vi "Finish.vi"   [LabVIEW 2017]
doc: "This VI is called just before exiting. It is expected to close I/O refnum, save collected data, etc."
uses:
  <vilib>/Rock Robotics/WPI/Utilities/WPI_GetSetVariantRefNum.vi
types:
  T1 = typedef "WPI_MotorControlDeviceRef.ctl" = cluster{"DeviceStatus":errorcluster, "Type":T2, "PWM":cluster{"PWM Channel":T3, "DeadBand":T4}, "CAN":cluster{"Device Number":u8, "SetOutput VI Ref":variant, "GetOutput VI Ref":variant, "Enable VI Ref":variant, "Disable VI Ref":variant, "Data":variant}, "Invert":bool, "DIO PWM":cluster{"PWM \"Enable\" Channel":T3, "DIOChannel":T5, "PWM Rate":dbl}}
  T2 = typedef "WPI_MotorControlType.ctl" = enum16{"PWM", "CAN", "DIO PWM"}
  T3 = typedef "FPGA_DIOPWMChannel.ctl" = enum8{"PWM 0", "PWM 1", "PWM 2", "PWM 3", "PWM 4", "PWM 5", "PWM 6", "PWM 7", "PWM 8", "PWM 9", "PWM MXP 0", "PWM MXP 1", "PWM MXP 2", "PWM MXP 3", "PWM MXP 4", "PWM MXP 5", "PWM MXP 6", "PWM MXP 7", "PWM MXP 8", "PWM MXP 9", "Invalid"}
  T4 = typedef "WPI_PWMDeadband.ctl" = cluster{"Name":string, "maxPositivePwm":i32, "minPositivePwm":i32, "centerPwm":i32, "maxNegativePwm":i32, "minNegativePwm":i32, "angularRange":u16}
  T5 = typedef "FPGA_DIOChannel.ctl" = enum8{"DIO 0", "DIO 1", "DIO 2", "DIO 3", "DIO 4", "DIO 5", "DIO 6", "DIO 7", "DIO 8", "DIO 9", "DIO MXP 0", "DIO MXP 1", "DIO MXP 2", "DIO MXP 3", "DIO MXP 4", "DIO MXP 5", "DIO MXP 6", "DIO MXP 7", "DIO MXP 8", "DIO MXP 9", "DIO MXP 10", "DIO MXP 11", "DIO MXP 12", "DIO MXP 13", "DIO MXP 14", "DIO MXP 15", "SPI Port CS1", "SPI Port CS2", "SPI Port CS3", "SPI Port MISO", "SPI Port MOSI", "Invalid"}
  T6 = typedef "WPI_JoystickDevRef.ctl" = cluster{"Device":T7}
  T7 = typedef "WPI_JoystickDeviceEnum.ctl" = enum16{"USB 0", "USB 1", "USB 2", "USB 3", "USB 4", "USB 5"}
  T8 = typedef "WPI_SolenoidDevRef.ctl" = cluster{"DevStatus":errorcluster, "Pneumatics Control Module":u8, "Forward Solenoid Channel":T9, "Reverse Solenoid Channel":T9}
  T9 = typedef "WPI_SolenoidChannel.ctl" = enum8{"Solenoid 0", "Solenoid 1", "Solenoid 2", "Solenoid 3", "Solenoid 4", "Solenoid 5", "Solenoid 6", "Solenoid 7", "Invalid"}
  T10 = typedef "WPI_EncoderDevRef.ctl" = cluster{"DevStatus":errorcluster, "EncoderIndex":T11, "CounterIndex":T12, "DistancePerCount":dbl, "Decoding Type":T13}
  T11 = typedef "FPGA_EncoderIdx.ctl" = enum8{"Enc 0", "Enc 1", "Enc 2", "Enc 3", "Enc 4", "Enc 5", "Enc 6", "Enc 7", "Invalid"}
  T12 = typedef "FPGA_CounterCtrSystemIndex.ctl" = enum8{"Ctr 0", "Ctr 1", "Ctr 2", "Ctr 3", "Ctr 4", "Ctr 5", "Ctr 6", "Ctr 7", "Invalid"}
  T13 = typedef "WPI_EncoderType.ctl" = enum16{"1x", "2x", "4x"}
  T14 = typedef "WPI_SwitchDevRef.ctl" = cluster{"DevStatus":errorcluster, "DIO Channel":T5, "CntIndex":T12, "Normally Closed":bool}
  T15 = typedef "WPI_CompressorDevRef.ctl" = cluster{"DevStatus":errorcluster, "Pneumatics Control Module":u8}
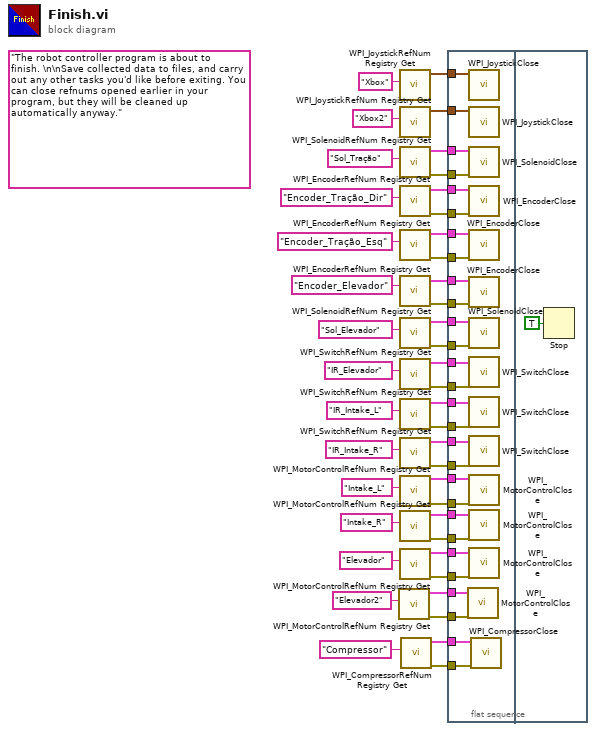
[diagram p0: block diagram]
diagram:
  (unwired) "The robot controller program is about to finish. \n\nSave collected data to files, and carry out any other tasks you'd like before exiting. You can close refnums opened earlier in your program, but they will be cleaned up automatically anyway."
  n1 = call <vilib>:"WPI_MotorControlRefNum Registry Get.vi"("refnum name"="Elevador2") -> ("error out"=w4:errorcluster, "MotorControlDevRef"=w5:T1)  [unwired: 9 in]
  n2 = call <vilib>:"WPI_JoystickRefNum Registry Get.vi"("refnum name"="Xbox") -> ("JoystickDevRef"=w43:T6)  [unwired: 9 in, 1 out]
  n3 = call <vilib>:"WPI_JoystickRefNum Registry Get.vi"("refnum name"="Xbox2") -> ("JoystickDevRef"=w42:T6)  [unwired: 9 in, 1 out]
  n4 = call <vilib>:"WPI_SolenoidRefNum Registry Get.vi"("refnum name"="Sol_Tração") -> ("error out"=w38:errorcluster, "SolenoidDevRef"=w39:T8)  [unwired: 9 in]
  n5 = call <vilib>:"WPI_EncoderRefNum Registry Get.vi"("refnum name"="Encoder_Tração_Dir") -> ("error out"=w35:errorcluster, "EncoderDevRef"=w36:T10)  [unwired: 9 in]
  n6 = call <vilib>:"WPI_EncoderRefNum Registry Get.vi"("refnum name"="Encoder_Tração_Esq") -> ("error out"=w11:errorcluster, "EncoderDevRef"=w10:T10)  [unwired: 9 in]
  n7 = call <vilib>:"WPI_EncoderRefNum Registry Get.vi"("refnum name"="Encoder_Elevador") -> ("error out"=w8:errorcluster, "EncoderDevRef"=w9:T10)  [unwired: 9 in]
  n8 = call <vilib>:"WPI_SolenoidRefNum Registry Get.vi"("refnum name"="Sol_Elevador") -> ("error out"=w33:errorcluster, "SolenoidDevRef"=w32:T8)  [unwired: 9 in]
  n9 = call <vilib>:"WPI_SwitchRefNum Registry Get.vi"("refnum name"="IR_Elevador") -> ("error out"=w29:errorcluster, "SwitchDevRef"=w30:T14)  [unwired: 9 in]
  n10 = call <vilib>:"WPI_SwitchRefNum Registry Get.vi"("refnum name"="IR_Intake_L") -> ("error out"=w27:errorcluster, "SwitchDevRef"=w26:T14)  [unwired: 9 in]
  n11 = call <vilib>:"WPI_SwitchRefNum Registry Get.vi"("refnum name"="IR_Intake_R") -> ("error out"=w24:errorcluster, "SwitchDevRef"=w25:T14)  [unwired: 9 in]
  n12 = call <vilib>:"WPI_MotorControlRefNum Registry Get.vi"("refnum name"="Intake_L") -> ("error out"=w20:errorcluster, "MotorControlDevRef"=w21:T1)  [unwired: 9 in]
  n13 = call <vilib>:"WPI_MotorControlRefNum Registry Get.vi"("refnum name"="Intake_R") -> ("error out"=w19:errorcluster, "MotorControlDevRef"=w18:T1)  [unwired: 9 in]
  n14 = call <vilib>:"WPI_MotorControlRefNum Registry Get.vi"("refnum name"="Elevador") -> ("error out"=w15:errorcluster, "MotorControlDevRef"=w14:T1)  [unwired: 9 in]
  n15 = call <vilib>:"WPI_CompressorRefNum Registry Get.vi"("refnum name"="Compressor") -> ("error out"=w1:errorcluster, "CompressorDevRef"=w2:T15)  [unwired: 9 in]
  n16 = flat-sequence {
    tunnel: w43 -> [w71]
    tunnel: w42 -> [w70]
    tunnel: w39 -> [w69]
    tunnel: w38 -> [w68]
    tunnel: w36 -> [w67]
    tunnel: w35 -> [w66]
    tunnel: w32 -> [w64]
    tunnel: w33 -> [w65]
    tunnel: w30 -> [w63]
    tunnel: w29 -> [w62]
    tunnel: w26 -> [w60]
    tunnel: w27 -> [w61]
    tunnel: w25 -> [w59]
    tunnel: w24 -> [w58]
    tunnel: w21 -> [w57]
    tunnel: w20 -> [w56]
    tunnel: w19 -> [w55]
    tunnel: w18 -> [w54]
    tunnel: w15 -> [w53]
    tunnel: w14 -> [w52]
    tunnel: w10 -> [w50]
    tunnel: w11 -> [w51]
    tunnel: w9 -> [w49]
    tunnel: w8 -> [w48]
    tunnel: w4 -> [w46]
    tunnel: w5 -> [w47]
    tunnel: w2 -> [w45]
    tunnel: w1 -> [w44]
    frame #0 {
      n17 = call <vilib>:"WPI_MotorControlClose.vi"("error in"=w46, "MotorControlDevRef"=w47) -> ()  [unwired: 9 in, 1 out]
      n18 = call <vilib>:"WPI_JoystickClose.vi"("JoystickDevRef"=w71) -> ()  [unwired: 11 in]
      n19 = call <vilib>:"WPI_JoystickClose.vi"("JoystickDevRef"=w70) -> ()  [unwired: 11 in]
      n20 = call <vilib>:"WPI_SolenoidClose.vi"("error in (no error)"=w68, "SolenoidDevRef"=w69) -> ()  [unwired: 9 in, 1 out]
      n21 = call <vilib>:"WPI_EncoderClose.vi"("error in (no error)"=w66, "EncoderDevRef"=w67) -> ()  [unwired: 9 in, 1 out]
      n22 = call <vilib>:"WPI_EncoderClose.vi"("error in (no error)"=w51, "EncoderDevRef"=w50) -> ()  [unwired: 9 in, 1 out]
      n23 = call <vilib>:"WPI_EncoderClose.vi"("error in (no error)"=w48, "EncoderDevRef"=w49) -> ()  [unwired: 9 in, 1 out]
      n24 = call <vilib>:"WPI_SolenoidClose.vi"("error in (no error)"=w65, "SolenoidDevRef"=w64) -> ()  [unwired: 9 in, 1 out]
      n25 = call <vilib>:"WPI_SwitchClose.vi"("error in (no error)"=w62, "SwitchDevRef"=w63) -> ()  [unwired: 9 in, 1 out]
      n26 = call <vilib>:"WPI_SwitchClose.vi"("error in (no error)"=w61, "SwitchDevRef"=w60) -> ()  [unwired: 9 in, 1 out]
      n27 = call <vilib>:"WPI_SwitchClose.vi"("error in (no error)"=w58, "SwitchDevRef"=w59) -> ()  [unwired: 9 in, 1 out]
      n28 = call <vilib>:"WPI_MotorControlClose.vi"("error in"=w56, "MotorControlDevRef"=w57) -> ()  [unwired: 9 in, 1 out]
      n29 = call <vilib>:"WPI_MotorControlClose.vi"("error in"=w55, "MotorControlDevRef"=w54) -> ()  [unwired: 9 in, 1 out]
      n30 = call <vilib>:"WPI_MotorControlClose.vi"("error in"=w53, "MotorControlDevRef"=w52) -> ()  [unwired: 9 in, 1 out]
      n31 = call <vilib>:"WPI_CompressorClose.vi"("error in (no error)"=w44, "CompressorDevRef"=w45) -> ()  [unwired: 9 in, 1 out]
    }
    frame #1 {
      n32 = Stop(stop? (T)=TRUE ("Quit")) -> ()
    }
  }
